vi "andrew_luis_sim.vi"() -> ()   [LabVIEW 2011]
panel:
  in  "Tab Control":T1(tab)
  in  "Initial Boat Location (x)":dbl=10.0
  in  "Initial Boat Location (y)":dbl=10.0
  in  "Waypoint Location (x)":dbl=16.0
  in  "Waypoint Location (y)":dbl=16.0
  in  "Absolute Wind Dir":i32(knob)=45 scale=-180.0..180.0
  in  "Initial Boat Heading":i32(knob) scale=-180.0..180.0
  in  "Loop delay (ms)":u32=100
  in  "v*dt":dbl=0.1
  out "Loop Iteration":i32
  out "Boat Path":cluster{"X":dbl, "Y":dbl}[](graph)
  out "Boat Location (y)":dbl
  out "Boat Location (x)":dbl
  out "Absolute heading\ntowards wpt":dbl
  out "dx and dy":cluster{"X":dbl, "Y":dbl}
  out "Distance to waypt":cluster{"X":dbl, "Y":dbl}
  out "New heading":i32(knob) scale=-180.0..180.0
  out "Apparent Wind Dir":i32(knob) scale=-180.0..180.0
  out "Last Heading":i32
  in  "stop":bool
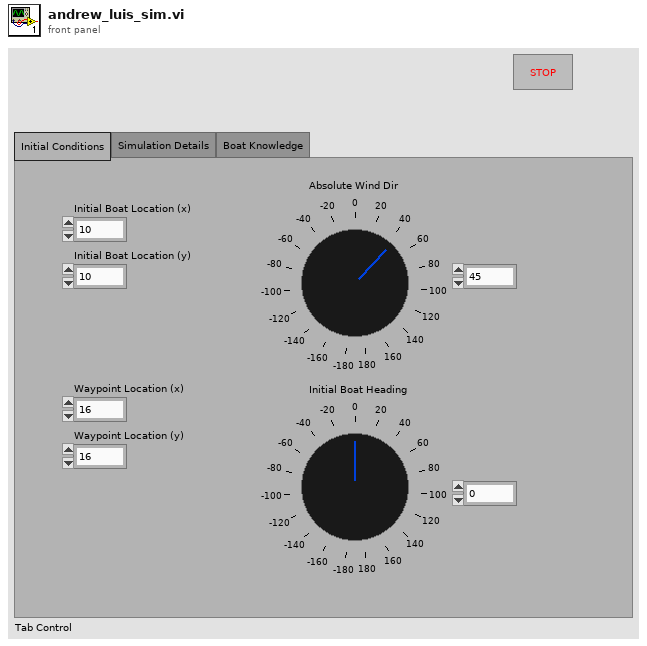
[diagram p1: front panel]
types:
  T1 = enum32{"Initial Conditions", "Simulation Details", "Boat Knowledge"}
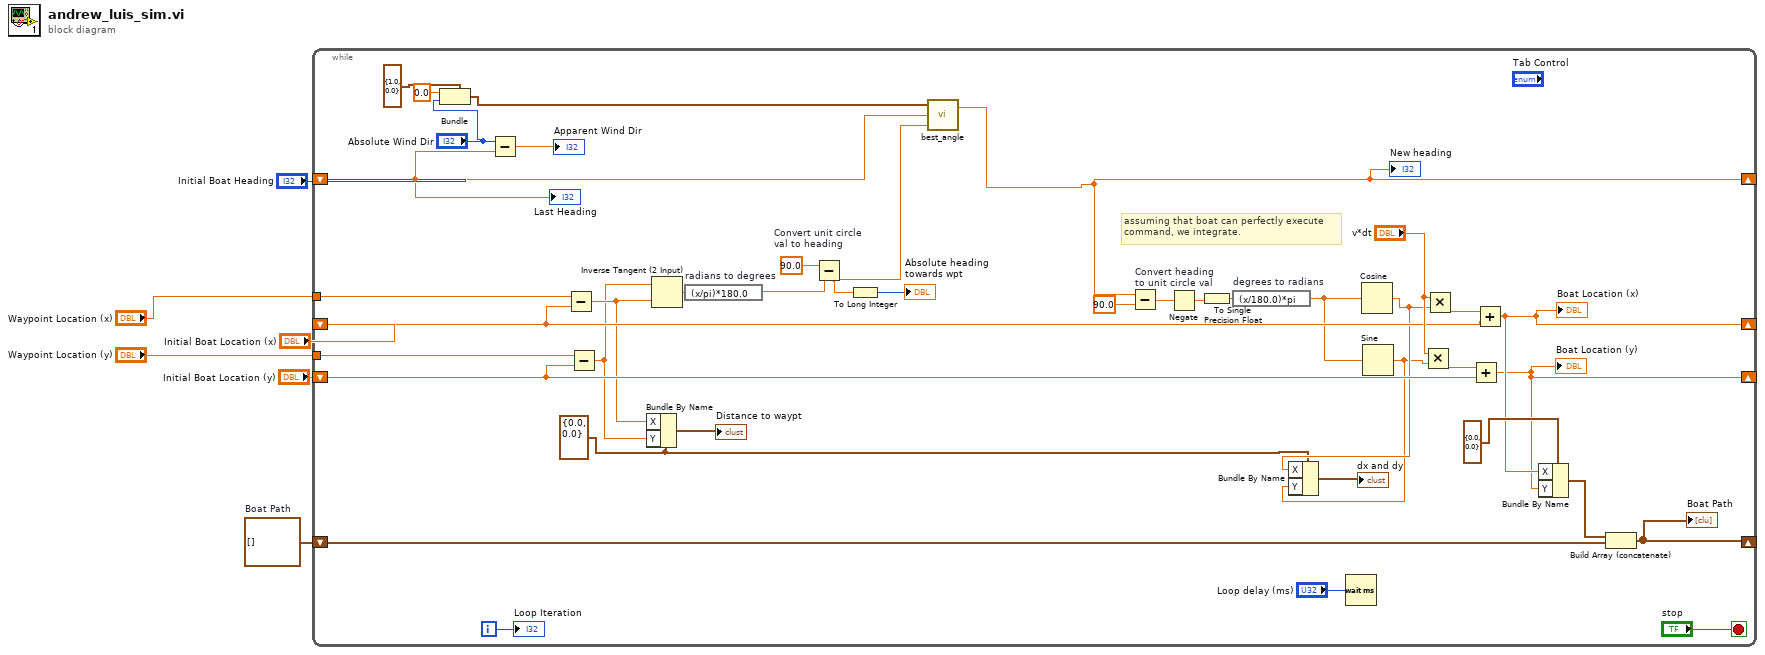
[diagram p0: block diagram]
diagram:
  w1 = cluster{"X":dbl, "Y":dbl}[] []  # Boat Path
  n1 = while {
    shift-right: [w37] -> _
    shift-left: "Initial Boat Location (x)" -> [w40]
    shift-right: [w36] -> _
    shift-left: "Initial Boat Location (y)" -> [w39]
    tunnel: "Waypoint Location (x)" -> [w42]
    tunnel: "Waypoint Location (y)" -> [w41]
    shift-right: [w9] -> _
    shift-left: "Initial Boat Heading" -> [w14]
    shift-right: [w34] -> _
    shift-left: w1 -> [w33]
    i -> [w32]
    stop <- "stop" stop-if-true
    w24 = cluster{"X":dbl, "Y":dbl} {"X"=0.0, "Y"=0.0} ("Cluster")
    # "assuming that boat can perfectly execute\ncommand, we integrate."
    n2 = Bundle(cluster=cluster{"Wind R":dbl, "Wind Theta":dbl} {"Wind R"=1.0, "Wind Theta"=0.0} ("Wind Vector"), "Wind R"=0.0, "Wind Theta"="Absolute Wind Dir") -> (w13:cluster{"Wind R":dbl, "Wind Theta":dbl})
    n3 = Subtract(x="Absolute Wind Dir", y=w14) -> (x-y=→"Apparent Wind Dir":dbl)
    n4 = Subtract(x=w42, y=w40) -> (x-y=w22:dbl)
    n5 = Subtract(x=w41, y=w39) -> (x-y=w21:dbl)
    n6 = Bundle By Name(cluster=w24, "X"=w22, "Y"=w21) -> (→"Distance to waypt":cluster{"X":dbl, "Y":dbl})
    n7 = Inverse Tangent (2 Input)(1:w22, 2:w21) -> (0:w23:dbl)
    n8 = expression code="(x/pi)*180.0" "radians to degrees"(w23) -> (w20:dbl)
    n9 = Subtract "Convert unit circle\nval to heading"(x=90.0, y=w20) -> (x-y=w8:dbl)
    n10 = To Long Integer(number=w8) -> (32bit integer=→"Absolute heading\ntowards wpt":i32)
    n11 = call "best_angle.vi"("Waypoint Heading"=w8, "Current Heading"=w14, "Wind Vector"=w13) -> ("Best Angle"=w9:dbl)  [unwired: 1 in]
    "New heading" <- w9
    n12 = Subtract "Convert heading \nto unit circle val"(x=w9, y=90.0 ("x")) -> (x-y=w16:dbl)
    n13 = Negate(x=w16) -> (-x=w17:dbl)
    n14 = To Single Precision Float(number=w17) -> (single precision float=w28:sgl)
    n15 = expression code="(x/180.0)*pi" "degrees to radians"(w28) -> (w29:sgl)
    n16 = Wait (ms)(milliseconds to wait="Loop delay (ms)") -> ()  [unwired: 1 out]
    n17 = Cosine(x=w29) -> (cos(x)=w26:sgl)
    n18 = Sine(x=w29) -> (sin(x)=w25:sgl)
    n19 = Bundle By Name(cluster=w24, "X"=w26, "Y"=w25) -> (→"dx and dy":cluster{"X":dbl, "Y":dbl})
    n20 = Multiply(x="v*dt", y=w25) -> (x*y=w45:dbl)
    n21 = Multiply(x="v*dt", y=w26) -> (x*y=w44:dbl)
    n22 = Add(x=w45, y=w39) -> (x+y=w36:dbl)
    "Boat Location (y)" <- w36
    n23 = Add(x=w44, y=w40) -> (x+y=w37:dbl)
    "Boat Location (x)" <- w37
    n24 = Bundle By Name(cluster=cluster{"X":dbl, "Y":dbl} {"X"=0.0, "Y"=0.0}, "X"=w37, "Y"=w36) -> (w35:cluster{"X":dbl, "Y":dbl})
    n25 = Build Array (concatenate)(w35, w33) -> (w34:cluster{"X":dbl, "Y":dbl}[])
    "Boat Path" <- w34
    "Loop Iteration" <- w32
    "Last Heading" <- w14
  }
